vi "Send_FirmwareUpgrade_Cmd_SUB_VI.vi"(4 "Message Length":i32, 7 "Which one to upgrade? AC||PC||SC":string="1||1||1", 8 "Error Input":errorcluster, 9 "Message ID":i32, 10 "Response ID":i32, 11 "TCP_IN":refnum<k5>) -> (0 "Error Out put":errorcluster, 3 "FW Upgrade Results":string)   [LabVIEW 2017]
panel:
  out "connection ID out":refnum<k5>
  # "INPUT :"
  # "INPUT :"
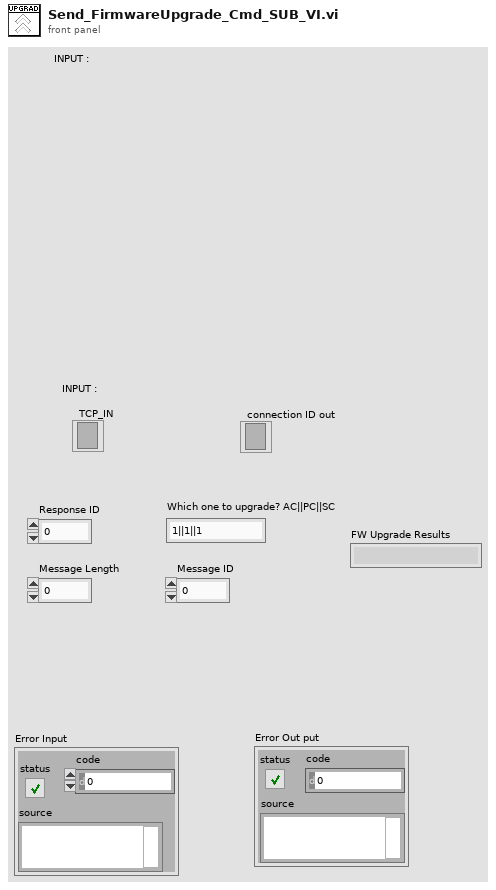
[diagram p1: front panel]
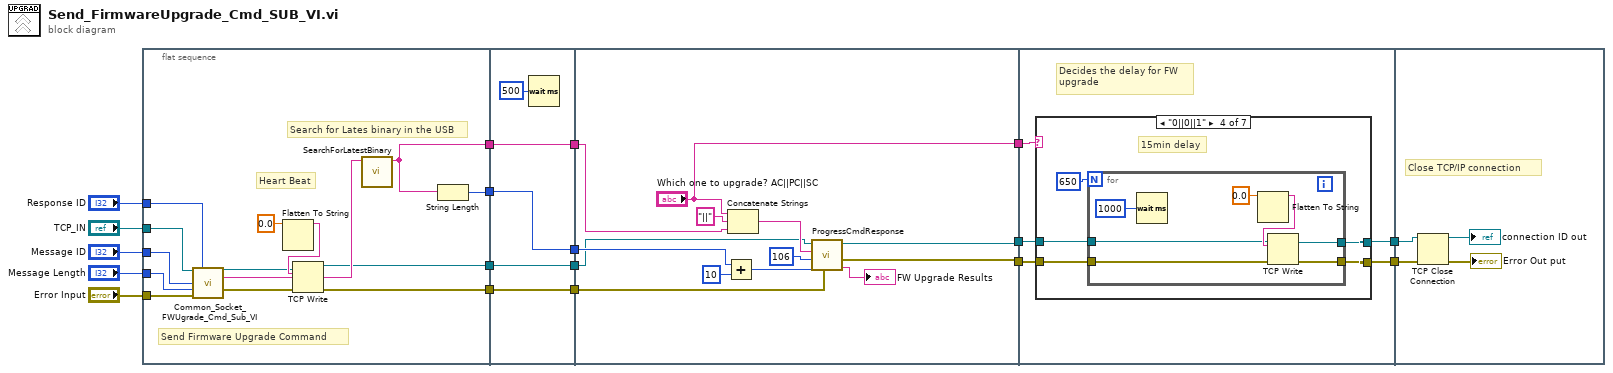
[diagram p0: block diagram]
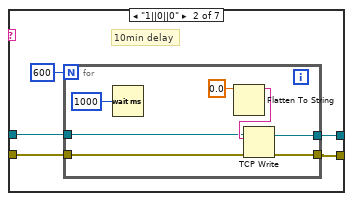
[diagram p3: hidden frame]
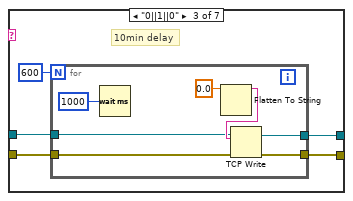
[diagram p4: hidden frame]
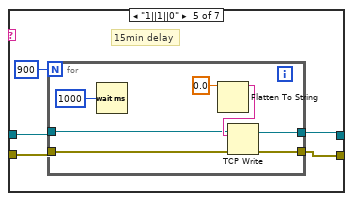
[diagram p5: hidden frame]
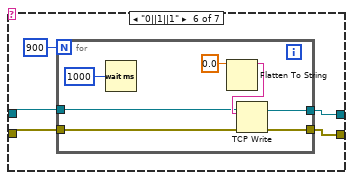
[diagram p6: hidden frame]
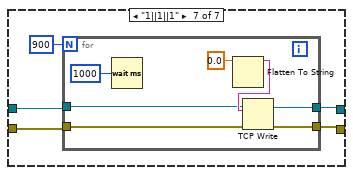
[diagram p7: hidden frame]
diagram:
  n1 = flat-sequence {
    tunnel: [w23] -> w10
    tunnel: [w26] -> w8
    tunnel: "Message ID" -> [w31]
    tunnel: "Response ID" -> [w32]
    tunnel: "Message Length" -> [w30]
    tunnel: "Error Input" -> [w29]
    tunnel: [w27] -> w5
    tunnel: "TCP_IN" -> [w20]
    tunnel: [w19] -> w1
    tunnel: w10 -> [w37]
    tunnel: [w37] -> w9
    tunnel: w8 -> [w36]
    tunnel: [w36] -> w7
    tunnel: [w34] -> w6
    tunnel: w5 -> [w34]
    tunnel: [w33] -> w2
    tunnel: w1 -> [w33]
    tunnel: w9 -> [w48]
    tunnel: w7 -> [w50]
    tunnel: [w46] -> w12
    tunnel: [w45] -> w11
    tunnel: w6 -> [w39]
    tunnel: ["Which one to upgrade? AC||PC||SC"] -> w4
    tunnel: w2 -> [w38]
    tunnel: [w52] -> w18
    tunnel: [w51] -> w17
    tunnel: w12 -> [w54]
    tunnel: w11 -> [w53]
    tunnel: w4 -> [w55]
    tunnel: w18 -> [w132]
    tunnel: w17 -> [w131]
    frame #0 {
      # "Heart Beat"
      # "Search for Lates binary in the USB"
      # "Send Firmware Upgrade Command"
      n2 = call "Common_Socket_FWUgrade_Cmd_Sub_VI.vi"("TCP_IN"=w20, "Response ID 1"=w32, "FW Message ID"=w31, "FW Message Length"=w30, "error in"=w29) -> ("connection ID"=w21:refnum<k5>, "Data Response"=w28:string, "error out"=w22:errorcluster)  [unwired: 7 in, 1 out]
      n3 = Flatten To String(anything=0.0) -> (data string=w24:string)  [unwired: 3 in, 2 out]
      n4 = TCP Write(connection ID=w21, data in=w24, error in (no error)=w22) -> (connection ID out=w19:refnum<k5>, error out=w23:errorcluster)  [unwired: 1 in, 1 out]
      n5 = call "SearchForLatestBinary.vi"("Input string"=w28) -> ("Output string"=w26:string)  [unwired: 10 in]
      n6 = String Length(string=w26) -> (length=w27:i32)
    }
    frame #1 {
      n7 = Wait (ms)(milliseconds to wait=u32 500) -> ()  [unwired: 1 out]
    }
    frame #2 {
      n8 = Add(x=w39, y=10) -> (x+y=w42:i32)
      n9 = Concatenate Strings("Which one to upgrade? AC||PC||SC", "||" ("string"), w50) -> (w44:string)
      n10 = call "ProgressCmdResponse.vi"("error in (no error)"=w48, "FW Message Length"=w42, "FW Message ID"=106, "Command for FW upgrade"=w44, "connection ID control"=w38) -> ("data out"=→"FW Upgrade Results":string, "error out"=w45:errorcluster, "connection ID"=w46:refnum<k5>)  [unwired: 4 in]
    }
    frame #3 {
      # "Decides the delay for FW \nupgrade"
      n11 = case shown="\"0||0||1\"" w55 {
        tunnel: w54 -> [w57 w61 w74 w86 w98 w110 w122]
        tunnel: w53 -> [w56 w60 w73 w85 w97 w109 w121]
        tunnel: [w57 w59 w72 w84 w96 w108 w120] -> w52
        tunnel: [w56 w58 w71 w83 w95 w107 w119] -> w51
        frame "False", Default {
        }
        frame "1||0||0" {
          # "10min delay"
          n12 = for {
            N: 600 -> [_]
            tunnel: w61 -> [w66]
            tunnel: w60 -> [w65]
            tunnel: [w64] -> w59
            tunnel: [w63] -> w58
            n13 = Wait (ms)(milliseconds to wait=u32 1000) -> ()  [unwired: 1 out]
            n14 = Flatten To String(anything=0.0) -> (data string=w67:string)  [unwired: 3 in, 2 out]
            n15 = TCP Write(connection ID=w66, data in=w67, error in (no error)=w65) -> (connection ID out=w64:refnum<k5>, error out=w63:errorcluster)  [unwired: 1 in, 1 out]
          }
        }
        frame "0||1||0" {
          # "10min delay"
          n16 = for {
            N: 600 -> [_]
            tunnel: w74 -> [w78]
            tunnel: w73 -> [w77]
            tunnel: [w76] -> w72
            tunnel: [w75] -> w71
            n17 = Wait (ms)(milliseconds to wait=u32 1000) -> ()  [unwired: 1 out]
            n18 = Flatten To String(anything=0.0) -> (data string=w79:string)  [unwired: 3 in, 2 out]
            n19 = TCP Write(connection ID=w78, data in=w79, error in (no error)=w77) -> (connection ID out=w76:refnum<k5>, error out=w75:errorcluster)  [unwired: 1 in, 1 out]
          }
        }
        frame "0||0||1" {
          # "15min delay"
          n20 = for {
            N: 650 -> [_]
            tunnel: w86 -> [w90]
            tunnel: w85 -> [w89]
            tunnel: [w88] -> w84
            tunnel: [w87] -> w83
            n21 = Wait (ms)(milliseconds to wait=u32 1000) -> ()  [unwired: 1 out]
            n22 = Flatten To String(anything=0.0) -> (data string=w91:string)  [unwired: 3 in, 2 out]
            n23 = TCP Write(connection ID=w90, data in=w91, error in (no error)=w89) -> (connection ID out=w88:refnum<k5>, error out=w87:errorcluster)  [unwired: 1 in, 1 out]
          }
        }
        frame "1||1||0" {
          # "15min delay"
          n24 = for {
            N: 900 -> [_]
            tunnel: w98 -> [w102]
            tunnel: w97 -> [w101]
            tunnel: [w100] -> w96
            tunnel: [w99] -> w95
            n25 = Wait (ms)(milliseconds to wait=u32 1000) -> ()  [unwired: 1 out]
            n26 = Flatten To String(anything=0.0) -> (data string=w103:string)  [unwired: 3 in, 2 out]
            n27 = TCP Write(connection ID=w102, data in=w103, error in (no error)=w101) -> (connection ID out=w100:refnum<k5>, error out=w99:errorcluster)  [unwired: 1 in, 1 out]
          }
        }
        frame "0||1||1" {
          n28 = for {
            N: 900 -> [_]
            tunnel: w110 -> [w114]
            tunnel: w109 -> [w113]
            tunnel: [w112] -> w108
            tunnel: [w111] -> w107
            n29 = Wait (ms)(milliseconds to wait=u32 1000) -> ()  [unwired: 1 out]
            n30 = Flatten To String(anything=0.0) -> (data string=w115:string)  [unwired: 3 in, 2 out]
            n31 = TCP Write(connection ID=w114, data in=w115, error in (no error)=w113) -> (connection ID out=w112:refnum<k5>, error out=w111:errorcluster)  [unwired: 1 in, 1 out]
          }
        }
        frame "1||1||1" {
          n32 = for {
            N: 900 -> [_]
            tunnel: w122 -> [w126]
            tunnel: w121 -> [w125]
            tunnel: [w124] -> w120
            tunnel: [w123] -> w119
            n33 = Wait (ms)(milliseconds to wait=u32 1000) -> ()  [unwired: 1 out]
            n34 = Flatten To String(anything=0.0) -> (data string=w127:string)  [unwired: 3 in, 2 out]
            n35 = TCP Write(connection ID=w126, data in=w127, error in (no error)=w125) -> (connection ID out=w124:refnum<k5>, error out=w123:errorcluster)  [unwired: 1 in, 1 out]
          }
        }
      }
    }
    frame #4 {
      # "Close TCP/IP connection"
      n36 = TCP Close Connection(connection ID=w132, error in (no error)=w131) -> (connection ID out=→"connection ID out":refnum<k5>, error out=→"Error Out put":errorcluster)  [unwired: 1 in]
    }
  }
